vi "VideoIO GetWriterBackends.vi"(8 "error in":errorcluster) -> (0 "error out":errorcluster, 3 "Backends":T1[](array[typedef]) items=["CAP_ANY"=0, "CAP_VFW/CAP_V4L"=200, "CAP_FIREWIRE"=300, "CAP_QT"=500, "CAP_UNICAP"=600, "CAP_DSHOW"=700, "CAP_PVAPI"=800, "CAP_OPENNI"=900, "CAP_OPENNI_ASUS"=910, "CAP_ANDROID"=1000, "CAP_XIAPI"=1100, "CAP_AVFOUNDATION"=1200, "CAP_GIGANETIX"=1300, "CAP_MSMF"=1400, "CAP_WINRT"=1410, "CAP_INTELPERC/CAP_REALSENSE"=1500, "CAP_OPENNI2"=1600, "CAP_OPENNI2_ASUS"=1610, "CAP_OPENNI2_ASTRA"=1620, "CAP_GPHOTO2"=1700, "CAP_GSTREAMER"=1800, "CAP_FFMPEG"=1900, "CAP_IMAGES"=2000, "CAP_ARAVIS"=2100, "CAP_OPENCV_MJPEG"=2200, "CAP_INTEL_MFX"=2300, "CAP_XINE"=2400, "CAP_UEYE"=2500, "CAP_OBSENSOR"=2600])   [LabVIEW 2020, in "OpenLvVision_OpenCv.lvlib"]
doc: "eturns list of available backends which works via cv::VideoWriter()"
uses:
  OpenLvVision_OpenCv.lvlib
  TypeDef/VideoCaptureAPIs.ctl
  Dlls/OlvOpenCvWrapper.dll
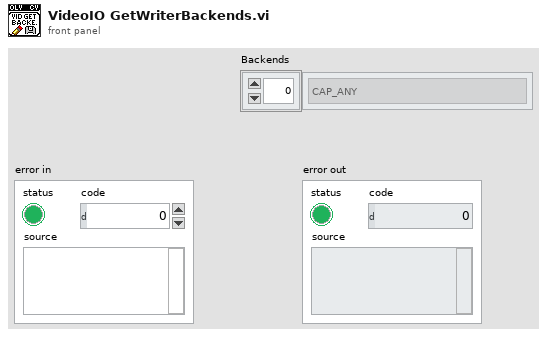
[diagram p1: front panel]
types:
  T1 = typedef "OpenLvVision_OpenCv.lvlib/VideoCaptureAPIs.ctl" = i32
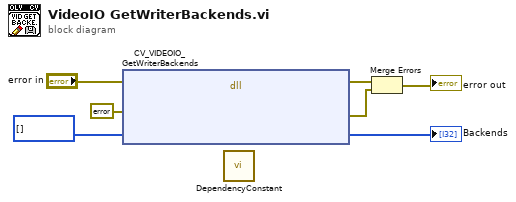
[diagram p0: block diagram]
diagram:
  w2 = T1[] [] items=["CAP_ANY"=0, "CAP_VFW/CAP_V4L"=200, "CAP_FIREWIRE"=300, "CAP_QT"=500, "CAP_UNICAP"=600, "CAP_DSHOW"=700, "CAP_PVAPI"=800, "CAP_OPENNI"=900, "CAP_OPENNI_ASUS"=910, "CAP_ANDROID"=1000, "CAP_XIAPI"=1100, "CAP_AVFOUNDATION"=1200, "CAP_GIGANETIX"=1300, "CAP_MSMF"=1400, "CAP_WINRT"=1410, "CAP_INTELPERC/CAP_REALSENSE"=1500, "CAP_OPENNI2"=1600, "CAP_OPENNI2_ASUS"=1610, "CAP_OPENNI2_ASTRA"=1620, "CAP_GPHOTO2"=1700, "CAP_GSTREAMER"=1800, "CAP_FFMPEG"=1900, "CAP_IMAGES"=2000, "CAP_ARAVIS"=2100, "CAP_OPENCV_MJPEG"=2200, "CAP_INTEL_MFX"=2300, "CAP_XINE"=2400, "CAP_UEYE"=2500, "CAP_OBSENSOR"=2600]
  n1 = dll-call lib="C:/Users/lukas/Downloads/OpenLvVision_OpenCv/SourceCode/LabView/OpenLvVision_OpenCv/Dlls/OlvOpenCvWrapper.dll" fn="CV_VIDEOIO_GetWriterBackends"(error in="error in", "Error"=errorcluster {"status"=FALSE, "code"=0, "source"=""} ("error out"), "backendArrayHandle"=w2) -> (error out=w6:errorcluster, "Error"=w4:errorcluster, "backendArrayHandle"=→"Backends":T1[])  [unwired: 3 in, 1 out]
  n2 = call "DependencyConstant.vi"() -> ()  [unwired: 12 in]
  n3 = Merge Errors(w6, w4) -> (→"error out":errorcluster)
